vi "real time object finder single cam 4 way v2.2 EJA 10 31 2016.vi"() -> ()   [LabVIEW 2013]
doc: "The Low-Level Grab VI acquires images continuously and displays the images in an image control using low-level acquisition VIs. A grab is appropriate for high-speed applications in which you need to process only one image at a time."
uses:
  <vilib>/userdefined/High Color/IMAQdx.ctl
  <vilib>/vision/driver/IMAQdx.llb/IMAQdx Buffer Number Mode.ctl
  <vilib>/Utility/file.llb/Write To Spreadsheet File (I64).vi
  <vilib>/vision/driver/NI_Vision_Acquisition_Software.lvlib
  <resource>/objmgr/imaqdx.rc
  <vilib>/Analysis/NI_AALBase.lvlib
panel:
  in  "Rectangle":T1
  in  "fish size":i32=200
  out "y position histogram":T2(graph)={"X Values"=[445.05, 445.15, 445.25, 445.35, 445.45, 445.55, 445.65, 445.75, 445.85, 445.95], "Histogram: h(x)"=[161, 0, 0, 0, 0, 0, 0, 0, 0, 90]}
  out "x position histogram":T2(graph)={"X Values"=[585.0, 585.0, 585.0, 585.0, 585.0, 585.0, 585.0, 585.0, 585.0, 585.0], "Histogram: h(x)"=[0, 0, 0, 0, 0, 0, 0, 0, 0, 251]}
  in  "histogram \nbins":i32=10
  in  "always save\non stop\nimaging":bool=TRUE
  in  "acquisition \ntime (s)":i32=5
  in  "save for a \ndesignated \nperiod":bool=TRUE
  out "trajectory":cluster{i32[], i32[]}(graph)={[585, 585, 585, 585, 585, 585, 585, 585, 585, 585, 585, 585, 585, 585, 585, 585, 585, 585, 585, 585, 585, 585, 585, 585, 585, 585, 585, 585, 585, 585, 585, 585, 585, 585, 585, 585, 585, 585, 585, 585, 585, 585, 585, 585, 585, 585, 585, 585, 585, 585, 585, 585, 585, 585, 585, 585, 585, 585, 585, 585, 585, 585, 585, 585, 585, 585, 585, 585, 585, 585, 585, 585, 585, 585, 585, 585, 585, 585, 585, 585, 585, 585, 585, 585, 585, 585, 585, 585, 585, 585, 585, 585, 585, 585, 585, 585, 585, 585, 585, 585, 585, 585, 585, 585, 585, 585, 585, 585, 585, 585, 585, 585, 585, 585, 585, 585, 585, 585, 585, 585, 585, 585, 585, 585, 585, 585, 585, 585, 585, 585, 585, 585, 585, 585, 585, 585, 585, 585, 585, 585, 585, 585, 585, 585, 585, 585, 585, 585, 585, 585, 585, 585, 585, 585, 585, 585, 585, 585, 585, 585, 585, 585, 585, 585, 585, 585, 585, 585, 585, 585, 585, 585, 585, 585, 585, 585, 585, 585, 585, 585, 585, 585, 585, 585, 585, 585, 585, 585, 585, 585, 585, 585, 585, 585, 585, 585, 585, 585, 585, 585, 585, 585, 585, 585, 585, 585, 585, 585, 585, 585, 585, 585, 585, 585, 585, 585, 585, 585, 585, 585, 585, 585, 585, 585, 585, 585, 585, 585, 585, 585, 585, 585, 585, 585, 585, 585, 585, 585, 585, 585, 585, 585, 585, 585, 585, 585, 585, 585, 585, 585, 585], [446, 446, 445, 445, 446, 445, 446, 445, 445, 445, 446, 445, 445, 446, 445, 445, 445, 446, 446, 445, 445, 446, 446, 445, 446, 445, 445, 445, 445, 445, 445, 445, 446, 446, 446, 445, 445, 446, 446, 446, 445, 445, 445, 445, 446, 446, 445, 445, 445, 446, 446, 446, 445, 446, 445, 445, 445, 445, 445, 445, 445, 446, 445, 445, 445, 445, 446, 445, 445, 445, 446, 445, 445, 445, 446, 446, 446, 445, 445, 445, 446, 446, 445, 445, 446, 445, 445, 446, 445, 445, 446, 445, 445, 445, 446, 446, 446, 445, 445, 445, 445, 445, 445, 446, 446, 446, 446, 445, 445, 445, 445, 446, 445, 446, 446, 445, 445, 445, 445, 446, 445, 445, 445, 446, 446, 446, 446, 446, 445, 445, 445, 446, 445, 445, 445, 445, 446, 445, 445, 445, 445, 445, 445, 446, 445, 446, 446, 446, 445, 445, 445, 445, 445, 446, 445, 446, 445, 445, 446, 445, 446, 445, 445, 445, 445, 445, 446, 446, 446, 446, 446, 445, 445, 446, 445, 445, 446, 445, 445, 445, 445, 446, 445, 445, 445, 445, 445, 445, 445, 446, 445, 445, 445, 446, 445, 445, 445, 446, 446, 445, 446, 445, 445, 446, 446, 445, 446, 445, 445, 445, 445, 445, 445, 445, 446, 445, 445, 445, 446, 445, 446, 445, 446, 446, 445, 446, 445, 445, 446, 446, 445, 445, 445, 446, 445, 445, 446, 445, 446, 445, 445, 445, 445, 446, 445, 445, 445, 445, 446, 445, 446]}
  in  "save\nlast\nimage":bool=TRUE
  in  "stop no save":bool
  out "date stub assigned":string="_2016Y_10M_31D_13h_38m_14s"
  in  "Acquire\ndata":bool
  in  "Experimental stub":string="danio02"
  out "Saving":bool
  in  "save data":bool
  in  "save path":path=path "C:/danio_tracking/danio02_10_28_2016"
  in  "number\nformat (%.6f)":string="%.6f"
  in  "Marker\nText color":u32(colorbox)=16711680
  out "Multiplot":cluster{cluster{dbl, i32}[]}[](graph)=[{[{0.0, 585}, {0.02, 585}, {0.04, 585}, {0.06, 585}, {0.08, 585}, {0.1, 585}, {0.12, 585}, {0.14, 585}, {0.16, 585}, {0.18, 585}, {0.2, 585}, {0.22, 585}, {0.24, 585}, {0.26, 585}, {0.28, 585}, {0.3, 585}, {0.32, 585}, {0.34, 585}, {0.36, 585}, {0.38, 585}, {0.4, 585}, {0.42, 585}, {0.44, 585}, {0.461, 585}, {0.48, 585}, {0.5, 585}, {0.52, 585}, {0.541, 585}, {0.561, 585}, {0.58, 585}, {0.601, 585}, {0.62, 585}, {0.641, 585}, {0.661, 585}, {0.681, 585}, {0.701, 585}, {0.721, 585}, {0.741, 585}, {0.761, 585}, {0.781, 585}, {0.801, 585}, {0.821, 585}, {0.841, 585}, {0.861, 585}, {0.881, 585}, {0.901, 585}, {0.921, 585}, {0.941, 585}, {0.961, 585}, {0.981, 585}, {1.001, 585}, {1.021, 585}, {1.041, 585}, {1.061, 585}, {1.082, 585}, {1.102, 585}, {1.122, 585}, {1.142, 585}, {1.162, 585}, {1.182, 585}, {1.202, 585}, {1.222, 585}, {1.242, 585}, {1.263, 585}, {1.282, 585}, {1.302, 585}, {1.322, 585}, {1.342, 585}, {1.363, 585}, {1.382, 585}, {1.402, 585}, {1.422, 585}, {1.442, 585}, {1.463, 585}, {1.482, 585}, {1.502, 585}, {1.522, 585}, {1.542, 585}, {1.563, 585}, {1.582, 585}, {1.602, 585}, {1.623, 585}, {1.642, 585}, {1.663, 585}, {1.682, 585}, {1.703, 585}, {1.723, 585}, {1.743, 585}, {1.763, 585}, {1.783, 585}, {1.803, 585}, {1.823, 585}, {1.843, 585}, {1.863, 585}, {1.883, 585}, {1.903, 585}, {1.923, 585}, {1.943, 585}, {1.963, 585}, {1.983, 585}, {2.003, 585}, {2.023, 585}, {2.043, 585}, {2.063, 585}, {2.083, 585}, {2.103, 585}, {2.123, 585}, {2.143, 585}, {2.163, 585}, {2.183, 585}, {2.203, 585}, {2.223, 585}, {2.243, 585}, {2.263, 585}, {2.283, 585}, {2.303, 585}, {2.323, 585}, {2.343, 585}, {2.363, 585}, {2.383, 585}, {2.403, 585}, {2.423, 585}, {2.443, 585}, {2.463, 585}, {2.484, 585}, {2.503, 585}, {2.524, 585}, {2.544, 585}, {2.564, 585}, {2.584, 585}, {2.604, 585}, {2.624, 585}, {2.644, 585}, {2.664, 585}, {2.684, 585}, {2.705, 585}, {2.725, 585}, {2.745, 585}, {2.765, 585}, {2.784, 585}, {2.805, 585}, {2.825, 585}, {2.845, 585}, {2.865, 585}, {2.885, 585}, {2.905, 585}, {2.925, 585}, {2.945, 585}, {2.965, 585}, {2.985, 585}, {3.005, 585}, {3.025, 585}, {3.045, 585}, {3.065, 585}, {3.085, 585}, {3.105, 585}, {3.125, 585}, {3.145, 585}, {3.165, 585}, {3.185, 585}, {3.205, 585}, {3.225, 585}, {3.245, 585}, {3.265, 585}, {3.285, 585}, {3.305, 585}, {3.325, 585}, {3.345, 585}, {3.365, 585}, {3.385, 585}, {3.405, 585}, {3.425, 585}, {3.445, 585}, {3.465, 585}, {3.485, 585}, {3.505, 585}, {3.525, 585}, {3.545, 585}, {3.565, 585}, {3.585, 585}, {3.605, 585}, {3.625, 585}, {3.646, 585}, {3.665, 585}, {3.685, 585}, {3.705, 585}, {3.725, 585}, {3.747, 585}, {3.765, 585}, {3.786, 585}, {3.805, 585}, {3.825, 585}, {3.846, 585}, {3.865, 585}, {3.885, 585}, {3.907, 585}, {3.927, 585}, {3.947, 585}, {3.967, 585}, {3.987, 585}, {4.007, 585}, {4.027, 585}, {4.047, 585}, {4.067, 585}, {4.087, 585}, {4.107, 585}, {4.127, 585}, {4.147, 585}, {4.167, 585}, {4.187, 585}, {4.207, 585}, {4.227, 585}, {4.247, 585}, {4.267, 585}, {4.287, 585}, {4.307, 585}, {4.327, 585}, {4.347, 585}, {4.367, 585}, {4.387, 585}, {4.407, 585}, {4.427, 585}, {4.447, 585}, {4.467, 585}, {4.487, 585}, {4.507, 585}, {4.527, 585}, {4.547, 585}, {4.567, 585}, {4.587, 585}, {4.607, 585}, {4.627, 585}, {4.647, 585}, {4.667, 585}, {4.687, 585}, {4.707, 585}, {4.727, 585}, {4.748, 585}, {4.767, 585}, {4.787, 585}, {4.807, 585}, {4.828, 585}, {4.848, 585}, {4.867, 585}, {4.887, 585}, {4.907, 585}, {4.927, 585}, {4.948, 585}, {4.967, 585}, {4.988, 585}, {5.008, 585}]}, {[{0.0, 446}, {0.02, 446}, {0.04, 445}, {0.06, 445}, {0.08, 446}, {0.1, 445}, {0.12, 446}, {0.14, 445}, {0.16, 445}, {0.18, 445}, {0.2, 446}, {0.22, 445}, {0.24, 445}, {0.26, 446}, {0.28, 445}, {0.3, 445}, {0.32, 445}, {0.34, 446}, {0.36, 446}, {0.38, 445}, {0.4, 445}, {0.42, 446}, {0.44, 446}, {0.461, 445}, {0.48, 446}, {0.5, 445}, {0.52, 445}, {0.541, 445}, {0.561, 445}, {0.58, 445}, {0.601, 445}, {0.62, 445}, {0.641, 446}, {0.661, 446}, {0.681, 446}, {0.701, 445}, {0.721, 445}, {0.741, 446}, {0.761, 446}, {0.781, 446}, {0.801, 445}, {0.821, 445}, {0.841, 445}, {0.861, 445}, {0.881, 446}, {0.901, 446}, {0.921, 445}, {0.941, 445}, {0.961, 445}, {0.981, 446}, {1.001, 446}, {1.021, 446}, {1.041, 445}, {1.061, 446}, {1.082, 445}, {1.102, 445}, {1.122, 445}, {1.142, 445}, {1.162, 445}, {1.182, 445}, {1.202, 445}, {1.222, 446}, {1.242, 445}, {1.263, 445}, {1.282, 445}, {1.302, 445}, {1.322, 446}, {1.342, 445}, {1.363, 445}, {1.382, 445}, {1.402, 446}, {1.422, 445}, {1.442, 445}, {1.463, 445}, {1.482, 446}, {1.502, 446}, {1.522, 446}, {1.542, 445}, {1.563, 445}, {1.582, 445}, {1.602, 446}, {1.623, 446}, {1.642, 445}, {1.663, 445}, {1.682, 446}, {1.703, 445}, {1.723, 445}, {1.743, 446}, {1.763, 445}, {1.783, 445}, {1.803, 446}, {1.823, 445}, {1.843, 445}, {1.863, 445}, {1.883, 446}, {1.903, 446}, {1.923, 446}, {1.943, 445}, {1.963, 445}, {1.983, 445}, {2.003, 445}, {2.023, 445}, {2.043, 445}, {2.063, 446}, {2.083, 446}, {2.103, 446}, {2.123, 446}, {2.143, 445}, {2.163, 445}, {2.183, 445}, {2.203, 445}, {2.223, 446}, {2.243, 445}, {2.263, 446}, {2.283, 446}, {2.303, 445}, {2.323, 445}, {2.343, 445}, {2.363, 445}, {2.383, 446}, {2.403, 445}, {2.423, 445}, {2.443, 445}, {2.463, 446}, {2.484, 446}, {2.503, 446}, {2.524, 446}, {2.544, 446}, {2.564, 445}, {2.584, 445}, {2.604, 445}, {2.624, 446}, {2.644, 445}, {2.664, 445}, {2.684, 445}, {2.705, 445}, {2.725, 446}, {2.745, 445}, {2.765, 445}, {2.784, 445}, {2.805, 445}, {2.825, 445}, {2.845, 445}, {2.865, 446}, {2.885, 445}, {2.905, 446}, {2.925, 446}, {2.945, 446}, {2.965, 445}, {2.985, 445}, {3.005, 445}, {3.025, 445}, {3.045, 445}, {3.065, 446}, {3.085, 445}, {3.105, 446}, {3.125, 445}, {3.145, 445}, {3.165, 446}, {3.185, 445}, {3.205, 446}, {3.225, 445}, {3.245, 445}, {3.265, 445}, {3.285, 445}, {3.305, 445}, {3.325, 446}, {3.345, 446}, {3.365, 446}, {3.385, 446}, {3.405, 446}, {3.425, 445}, {3.445, 445}, {3.465, 446}, {3.485, 445}, {3.505, 445}, {3.525, 446}, {3.545, 445}, {3.565, 445}, {3.585, 445}, {3.605, 445}, {3.625, 446}, {3.646, 445}, {3.665, 445}, {3.685, 445}, {3.705, 445}, {3.725, 445}, {3.747, 445}, {3.765, 445}, {3.786, 446}, {3.805, 445}, {3.825, 445}, {3.846, 445}, {3.865, 446}, {3.885, 445}, {3.907, 445}, {3.927, 445}, {3.947, 446}, {3.967, 446}, {3.987, 445}, {4.007, 446}, {4.027, 445}, {4.047, 445}, {4.067, 446}, {4.087, 446}, {4.107, 445}, {4.127, 446}, {4.147, 445}, {4.167, 445}, {4.187, 445}, {4.207, 445}, {4.227, 445}, {4.247, 445}, {4.267, 445}, {4.287, 446}, {4.307, 445}, {4.327, 445}, {4.347, 445}, {4.367, 446}, {4.387, 445}, {4.407, 446}, {4.427, 445}, {4.447, 446}, {4.467, 446}, {4.487, 445}, {4.507, 446}, {4.527, 445}, {4.547, 445}, {4.567, 446}, {4.587, 446}, {4.607, 445}, {4.627, 445}, {4.647, 445}, {4.667, 446}, {4.687, 445}, {4.707, 445}, {4.727, 446}, {4.748, 445}, {4.767, 446}, {4.787, 445}, {4.807, 445}, {4.828, 445}, {4.848, 445}, {4.867, 446}, {4.887, 445}, {4.907, 445}, {4.927, 445}, {4.948, 445}, {4.967, 446}, {4.988, 445}, {5.008, 446}]}]
  out "FPS":i32=50
  out "time (s)":dbl[](array[numeric])=[0.0, 0.02, 0.04, 0.06, 0.08, 0.1, 0.12, 0.14, 0.16, 0.18, 0.2, 0.22, 0.24, 0.26, 0.28, 0.3, 0.32, 0.34, 0.36, 0.38, 0.4, 0.42, 0.44, 0.461, 0.48, 0.5, 0.52, 0.541, 0.561, 0.58, 0.601, 0.62, 0.641, 0.661, 0.681, 0.701, 0.721, 0.741, 0.761, 0.781, 0.801, 0.821, 0.841, 0.861, 0.881, 0.901, 0.921, 0.941, 0.961, 0.981, 1.001, 1.021, 1.041, 1.061, 1.082, 1.102, 1.122, 1.142, 1.162, 1.182, 1.202, 1.222, 1.242, 1.263, 1.282, 1.302, 1.322, 1.342, 1.363, 1.382, 1.402, 1.422, 1.442, 1.463, 1.482, 1.502, 1.522, 1.542, 1.563, 1.582, 1.602, 1.623, 1.642, 1.663, 1.682, 1.703, 1.723, 1.743, 1.763, 1.783, 1.803, 1.823, 1.843, 1.863, 1.883, 1.903, 1.923, 1.943, 1.963, 1.983, 2.003, 2.023, 2.043, 2.063, 2.083, 2.103, 2.123, 2.143, 2.163, 2.183, 2.203, 2.223, 2.243, 2.263, 2.283, 2.303, 2.323, 2.343, 2.363, 2.383, 2.403, 2.423, 2.443, 2.463, 2.484, 2.503, 2.524, 2.544, 2.564, 2.584, 2.604, 2.624, 2.644, 2.664, 2.684, 2.705, 2.725, 2.745, 2.765, 2.784, 2.805, 2.825, 2.845, 2.865, 2.885, 2.905, 2.925, 2.945, 2.965, 2.985, 3.005, 3.025, 3.045, 3.065, 3.085, 3.105, 3.125, 3.145, 3.165, 3.185, 3.205, 3.225, 3.245, 3.265, 3.285, 3.305, 3.325, 3.345, 3.365, 3.385, 3.405, 3.425, 3.445, 3.465, 3.485, 3.505, 3.525, 3.545, 3.565, 3.585, 3.605, 3.625, 3.646, 3.665, 3.685, 3.705, 3.725, 3.747, 3.765, 3.786, 3.805, 3.825, 3.846, 3.865, 3.885, 3.907, 3.927, 3.947, 3.967, 3.987, 4.007, 4.027, 4.047, 4.067, 4.087, 4.107, 4.127, 4.147, 4.167, 4.187, 4.207, 4.227, 4.247, 4.267, 4.287, 4.307, 4.327, 4.347, 4.367, 4.387, 4.407, 4.427, 4.447, 4.467, 4.487, 4.507, 4.527, 4.547, 4.567, 4.587, 4.607, 4.627, 4.647, 4.667, 4.687, 4.707, 4.727, 4.748, 4.767, 4.787, 4.807, 4.828, 4.848, 4.867, 4.887, 4.907, 4.927, 4.948, 4.967, 4.988, 5.008] format="%.3f"
  in  "Origin":cluster{"X":i32, "Y":i32}
  out "Y position vs time":cluster{dbl[], i32[]}(graph)={[0.0, 0.02, 0.04, 0.06, 0.08, 0.1, 0.12, 0.14, 0.16, 0.18, 0.2, 0.22, 0.24, 0.26, 0.28, 0.3, 0.32, 0.34, 0.36, 0.38, 0.4, 0.42, 0.44, 0.461, 0.48, 0.5, 0.52, 0.541, 0.561, 0.58, 0.601, 0.62, 0.641, 0.661, 0.681, 0.701, 0.721, 0.741, 0.761, 0.781, 0.801, 0.821, 0.841, 0.861, 0.881, 0.901, 0.921, 0.941, 0.961, 0.981, 1.001, 1.021, 1.041, 1.061, 1.082, 1.102, 1.122, 1.142, 1.162, 1.182, 1.202, 1.222, 1.242, 1.263, 1.282, 1.302, 1.322, 1.342, 1.363, 1.382, 1.402, 1.422, 1.442, 1.463, 1.482, 1.502, 1.522, 1.542, 1.563, 1.582, 1.602, 1.623, 1.642, 1.663, 1.682, 1.703, 1.723, 1.743, 1.763, 1.783, 1.803, 1.823, 1.843, 1.863, 1.883, 1.903, 1.923, 1.943, 1.963, 1.983, 2.003, 2.023, 2.043, 2.063, 2.083, 2.103, 2.123, 2.143, 2.163, 2.183, 2.203, 2.223, 2.243, 2.263, 2.283, 2.303, 2.323, 2.343, 2.363, 2.383, 2.403, 2.423, 2.443, 2.463, 2.484, 2.503, 2.524, 2.544, 2.564, 2.584, 2.604, 2.624, 2.644, 2.664, 2.684, 2.705, 2.725, 2.745, 2.765, 2.784, 2.805, 2.825, 2.845, 2.865, 2.885, 2.905, 2.925, 2.945, 2.965, 2.985, 3.005, 3.025, 3.045, 3.065, 3.085, 3.105, 3.125, 3.145, 3.165, 3.185, 3.205, 3.225, 3.245, 3.265, 3.285, 3.305, 3.325, 3.345, 3.365, 3.385, 3.405, 3.425, 3.445, 3.465, 3.485, 3.505, 3.525, 3.545, 3.565, 3.585, 3.605, 3.625, 3.646, 3.665, 3.685, 3.705, 3.725, 3.747, 3.765, 3.786, 3.805, 3.825, 3.846, 3.865, 3.885, 3.907, 3.927, 3.947, 3.967, 3.987, 4.007, 4.027, 4.047, 4.067, 4.087, 4.107, 4.127, 4.147, 4.167, 4.187, 4.207, 4.227, 4.247, 4.267, 4.287, 4.307, 4.327, 4.347, 4.367, 4.387, 4.407, 4.427, 4.447, 4.467, 4.487, 4.507, 4.527, 4.547, 4.567, 4.587, 4.607, 4.627, 4.647, 4.667, 4.687, 4.707, 4.727, 4.748, 4.767, 4.787, 4.807, 4.828, 4.848, 4.867, 4.887, 4.907, 4.927, 4.948, 4.967, 4.988, 5.008], [446, 446, 445, 445, 446, 445, 446, 445, 445, 445, 446, 445, 445, 446, 445, 445, 445, 446, 446, 445, 445, 446, 446, 445, 446, 445, 445, 445, 445, 445, 445, 445, 446, 446, 446, 445, 445, 446, 446, 446, 445, 445, 445, 445, 446, 446, 445, 445, 445, 446, 446, 446, 445, 446, 445, 445, 445, 445, 445, 445, 445, 446, 445, 445, 445, 445, 446, 445, 445, 445, 446, 445, 445, 445, 446, 446, 446, 445, 445, 445, 446, 446, 445, 445, 446, 445, 445, 446, 445, 445, 446, 445, 445, 445, 446, 446, 446, 445, 445, 445, 445, 445, 445, 446, 446, 446, 446, 445, 445, 445, 445, 446, 445, 446, 446, 445, 445, 445, 445, 446, 445, 445, 445, 446, 446, 446, 446, 446, 445, 445, 445, 446, 445, 445, 445, 445, 446, 445, 445, 445, 445, 445, 445, 446, 445, 446, 446, 446, 445, 445, 445, 445, 445, 446, 445, 446, 445, 445, 446, 445, 446, 445, 445, 445, 445, 445, 446, 446, 446, 446, 446, 445, 445, 446, 445, 445, 446, 445, 445, 445, 445, 446, 445, 445, 445, 445, 445, 445, 445, 446, 445, 445, 445, 446, 445, 445, 445, 446, 446, 445, 446, 445, 445, 446, 446, 445, 446, 445, 445, 445, 445, 445, 445, 445, 446, 445, 445, 445, 446, 445, 446, 445, 446, 446, 445, 446, 445, 445, 446, 446, 445, 445, 445, 446, 445, 445, 446, 445, 446, 445, 445, 445, 445, 446, 445, 445, 445, 445, 446, 445, 446]}
  out "X position vs time":cluster{dbl[], i32[]}(graph)={[0.0, 0.02, 0.04, 0.06, 0.08, 0.1, 0.12, 0.14, 0.16, 0.18, 0.2, 0.22, 0.24, 0.26, 0.28, 0.3, 0.32, 0.34, 0.36, 0.38, 0.4, 0.42, 0.44, 0.461, 0.48, 0.5, 0.52, 0.541, 0.561, 0.58, 0.601, 0.62, 0.641, 0.661, 0.681, 0.701, 0.721, 0.741, 0.761, 0.781, 0.801, 0.821, 0.841, 0.861, 0.881, 0.901, 0.921, 0.941, 0.961, 0.981, 1.001, 1.021, 1.041, 1.061, 1.082, 1.102, 1.122, 1.142, 1.162, 1.182, 1.202, 1.222, 1.242, 1.263, 1.282, 1.302, 1.322, 1.342, 1.363, 1.382, 1.402, 1.422, 1.442, 1.463, 1.482, 1.502, 1.522, 1.542, 1.563, 1.582, 1.602, 1.623, 1.642, 1.663, 1.682, 1.703, 1.723, 1.743, 1.763, 1.783, 1.803, 1.823, 1.843, 1.863, 1.883, 1.903, 1.923, 1.943, 1.963, 1.983, 2.003, 2.023, 2.043, 2.063, 2.083, 2.103, 2.123, 2.143, 2.163, 2.183, 2.203, 2.223, 2.243, 2.263, 2.283, 2.303, 2.323, 2.343, 2.363, 2.383, 2.403, 2.423, 2.443, 2.463, 2.484, 2.503, 2.524, 2.544, 2.564, 2.584, 2.604, 2.624, 2.644, 2.664, 2.684, 2.705, 2.725, 2.745, 2.765, 2.784, 2.805, 2.825, 2.845, 2.865, 2.885, 2.905, 2.925, 2.945, 2.965, 2.985, 3.005, 3.025, 3.045, 3.065, 3.085, 3.105, 3.125, 3.145, 3.165, 3.185, 3.205, 3.225, 3.245, 3.265, 3.285, 3.305, 3.325, 3.345, 3.365, 3.385, 3.405, 3.425, 3.445, 3.465, 3.485, 3.505, 3.525, 3.545, 3.565, 3.585, 3.605, 3.625, 3.646, 3.665, 3.685, 3.705, 3.725, 3.747, 3.765, 3.786, 3.805, 3.825, 3.846, 3.865, 3.885, 3.907, 3.927, 3.947, 3.967, 3.987, 4.007, 4.027, 4.047, 4.067, 4.087, 4.107, 4.127, 4.147, 4.167, 4.187, 4.207, 4.227, 4.247, 4.267, 4.287, 4.307, 4.327, 4.347, 4.367, 4.387, 4.407, 4.427, 4.447, 4.467, 4.487, 4.507, 4.527, 4.547, 4.567, 4.587, 4.607, 4.627, 4.647, 4.667, 4.687, 4.707, 4.727, 4.748, 4.767, 4.787, 4.807, 4.828, 4.848, 4.867, 4.887, 4.907, 4.927, 4.948, 4.967, 4.988, 5.008], [585, 585, 585, 585, 585, 585, 585, 585, 585, 585, 585, 585, 585, 585, 585, 585, 585, 585, 585, 585, 585, 585, 585, 585, 585, 585, 585, 585, 585, 585, 585, 585, 585, 585, 585, 585, 585, 585, 585, 585, 585, 585, 585, 585, 585, 585, 585, 585, 585, 585, 585, 585, 585, 585, 585, 585, 585, 585, 585, 585, 585, 585, 585, 585, 585, 585, 585, 585, 585, 585, 585, 585, 585, 585, 585, 585, 585, 585, 585, 585, 585, 585, 585, 585, 585, 585, 585, 585, 585, 585, 585, 585, 585, 585, 585, 585, 585, 585, 585, 585, 585, 585, 585, 585, 585, 585, 585, 585, 585, 585, 585, 585, 585, 585, 585, 585, 585, 585, 585, 585, 585, 585, 585, 585, 585, 585, 585, 585, 585, 585, 585, 585, 585, 585, 585, 585, 585, 585, 585, 585, 585, 585, 585, 585, 585, 585, 585, 585, 585, 585, 585, 585, 585, 585, 585, 585, 585, 585, 585, 585, 585, 585, 585, 585, 585, 585, 585, 585, 585, 585, 585, 585, 585, 585, 585, 585, 585, 585, 585, 585, 585, 585, 585, 585, 585, 585, 585, 585, 585, 585, 585, 585, 585, 585, 585, 585, 585, 585, 585, 585, 585, 585, 585, 585, 585, 585, 585, 585, 585, 585, 585, 585, 585, 585, 585, 585, 585, 585, 585, 585, 585, 585, 585, 585, 585, 585, 585, 585, 585, 585, 585, 585, 585, 585, 585, 585, 585, 585, 585, 585, 585, 585, 585, 585, 585, 585, 585, 585, 585, 585, 585]}
  in  "Pixel intensity\nthreshold":i32=65
  in  "Row min":i32=136
  in  "Row max":i32=630
  in  "Column min":i32=120
  in  "Column max":i32=1027
  out "X positions\ncamera 1\n(image \ncoordinates)":i32[](array[numeric])=[585, 585, 585, 585, 585, 585, 585, 585, 585, 585, 585, 585, 585, 585, 585, 585, 585, 585, 585, 585, 585, 585, 585, 585, 585, 585, 585, 585, 585, 585, 585, 585, 585, 585, 585, 585, 585, 585, 585, 585, 585, 585, 585, 585, 585, 585, 585, 585, 585, 585, 585, 585, 585, 585, 585, 585, 585, 585, 585, 585, 585, 585, 585, 585, 585, 585, 585, 585, 585, 585, 585, 585, 585, 585, 585, 585, 585, 585, 585, 585, 585, 585, 585, 585, 585, 585, 585, 585, 585, 585, 585, 585, 585, 585, 585, 585, 585, 585, 585, 585, 585, 585, 585, 585, 585, 585, 585, 585, 585, 585, 585, 585, 585, 585, 585, 585, 585, 585, 585, 585, 585, 585, 585, 585, 585, 585, 585, 585, 585, 585, 585, 585, 585, 585, 585, 585, 585, 585, 585, 585, 585, 585, 585, 585, 585, 585, 585, 585, 585, 585, 585, 585, 585, 585, 585, 585, 585, 585, 585, 585, 585, 585, 585, 585, 585, 585, 585, 585, 585, 585, 585, 585, 585, 585, 585, 585, 585, 585, 585, 585, 585, 585, 585, 585, 585, 585, 585, 585, 585, 585, 585, 585, 585, 585, 585, 585, 585, 585, 585, 585, 585, 585, 585, 585, 585, 585, 585, 585, 585, 585, 585, 585, 585, 585, 585, 585, 585, 585, 585, 585, 585, 585, 585, 585, 585, 585, 585, 585, 585, 585, 585, 585, 585, 585, 585, 585, 585, 585, 585, 585, 585, 585, 585, 585, 585, 585, 585, 585, 585, 585, 585]
  out "Y positions camera 1 \n(image \ncoordinates)":i32[](array[numeric])=[446, 446, 445, 445, 446, 445, 446, 445, 445, 445, 446, 445, 445, 446, 445, 445, 445, 446, 446, 445, 445, 446, 446, 445, 446, 445, 445, 445, 445, 445, 445, 445, 446, 446, 446, 445, 445, 446, 446, 446, 445, 445, 445, 445, 446, 446, 445, 445, 445, 446, 446, 446, 445, 446, 445, 445, 445, 445, 445, 445, 445, 446, 445, 445, 445, 445, 446, 445, 445, 445, 446, 445, 445, 445, 446, 446, 446, 445, 445, 445, 446, 446, 445, 445, 446, 445, 445, 446, 445, 445, 446, 445, 445, 445, 446, 446, 446, 445, 445, 445, 445, 445, 445, 446, 446, 446, 446, 445, 445, 445, 445, 446, 445, 446, 446, 445, 445, 445, 445, 446, 445, 445, 445, 446, 446, 446, 446, 446, 445, 445, 445, 446, 445, 445, 445, 445, 446, 445, 445, 445, 445, 445, 445, 446, 445, 446, 446, 446, 445, 445, 445, 445, 445, 446, 445, 446, 445, 445, 446, 445, 446, 445, 445, 445, 445, 445, 446, 446, 446, 446, 446, 445, 445, 446, 445, 445, 446, 445, 445, 445, 445, 446, 445, 445, 445, 445, 445, 445, 445, 446, 445, 445, 445, 446, 445, 445, 445, 446, 446, 445, 446, 445, 445, 446, 446, 445, 446, 445, 445, 445, 445, 445, 445, 445, 446, 445, 445, 445, 446, 445, 446, 445, 446, 446, 445, 446, 445, 445, 446, 446, 445, 445, 445, 446, 445, 445, 446, 445, 446, 445, 445, 445, 445, 446, 445, 445, 445, 445, 446, 445, 446]
  out "LIVE":bool
  in  "stop":bool
  out "Camera backlog":i32(slide)=-1 scale=0.0..50.0
  in  "IMAQdx Device Camera":T3="cam2"
  in  "Buffers Camera 1":u32=50
  out "Image":T4(plugin-control)
  # "PROGRAM INFO\n\nThis program finds the\nfirst pixel below the \nuser threshold in\nthe user specified\nROI below"
  # "Camera search ROI"
  # "Data acquisition \nsettings"
  # "issues\n\nHow do we know if frames \nare dropped?\n\nProbably will need to save data\nin sections to an open file\n\nCould have a sliding ROI based\non previous trailing edge position\n\nCould process each data chunk\nseparately to avoid frame dropping\nissues.  I.e. if you write every 1000\npoints, then in post processing only\nprocess 1000 at a time."
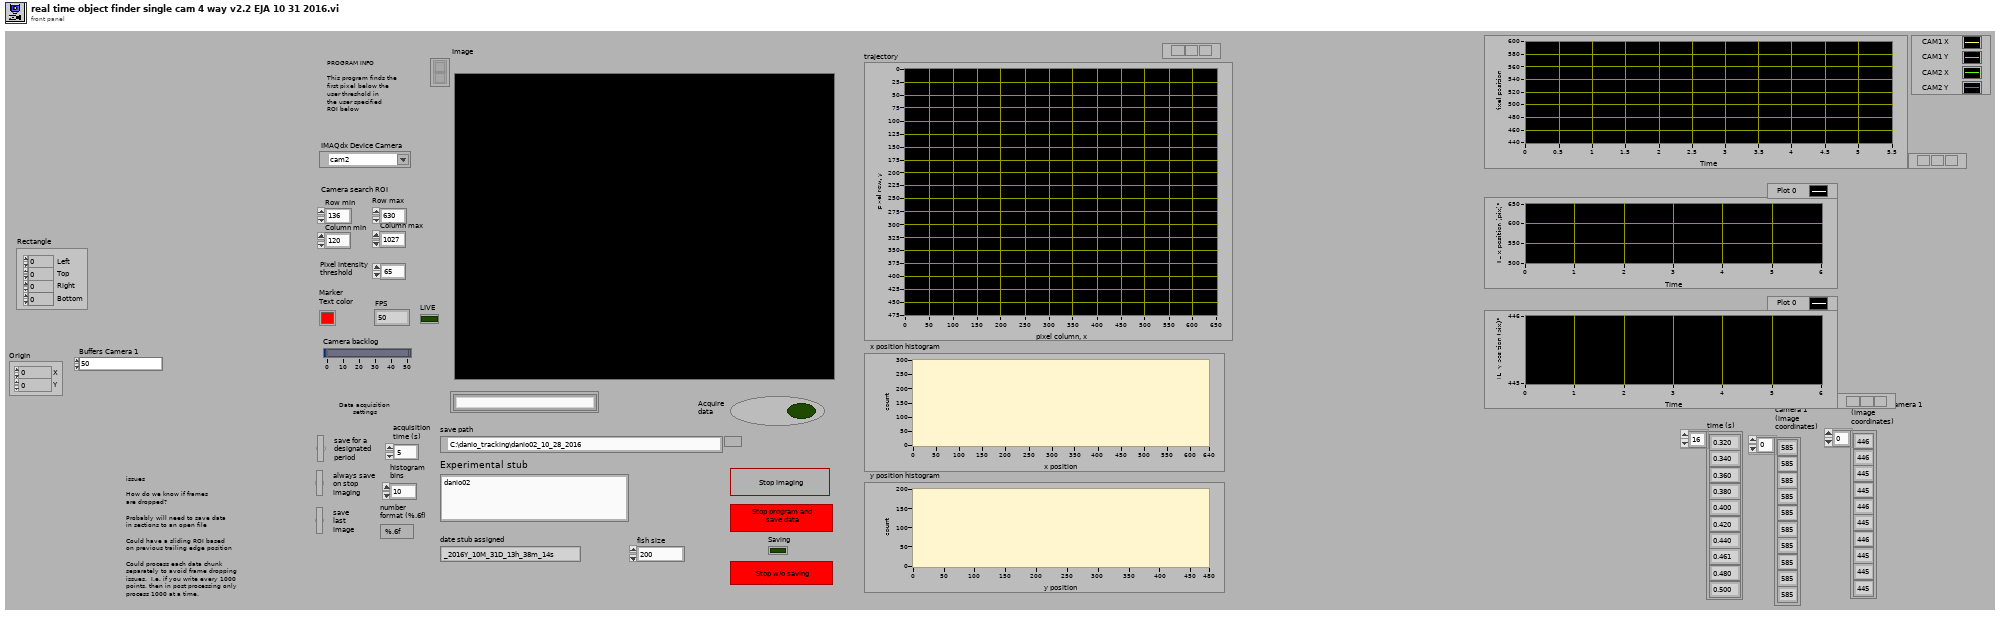
[diagram p1: front panel]
types:
  T1 = cluster{"Left":i32, "Top":i32, "Right":i32, "Bottom":i32}
  T2 = cluster{"X Values":dbl[], "Histogram: h(x)":i32[]}
  T3 = typedef "IMAQdx.ctl" = refnum<k21>
  T4 = typedef "IMAQ Image.ctl" = refnum<image>
  T5 = typedef "NI_Vision_Acquisition_Software.lvlib/IMAQdx Buffer Number Mode.ctl" = enum32{"Next", "Last", "Buffer Number"}
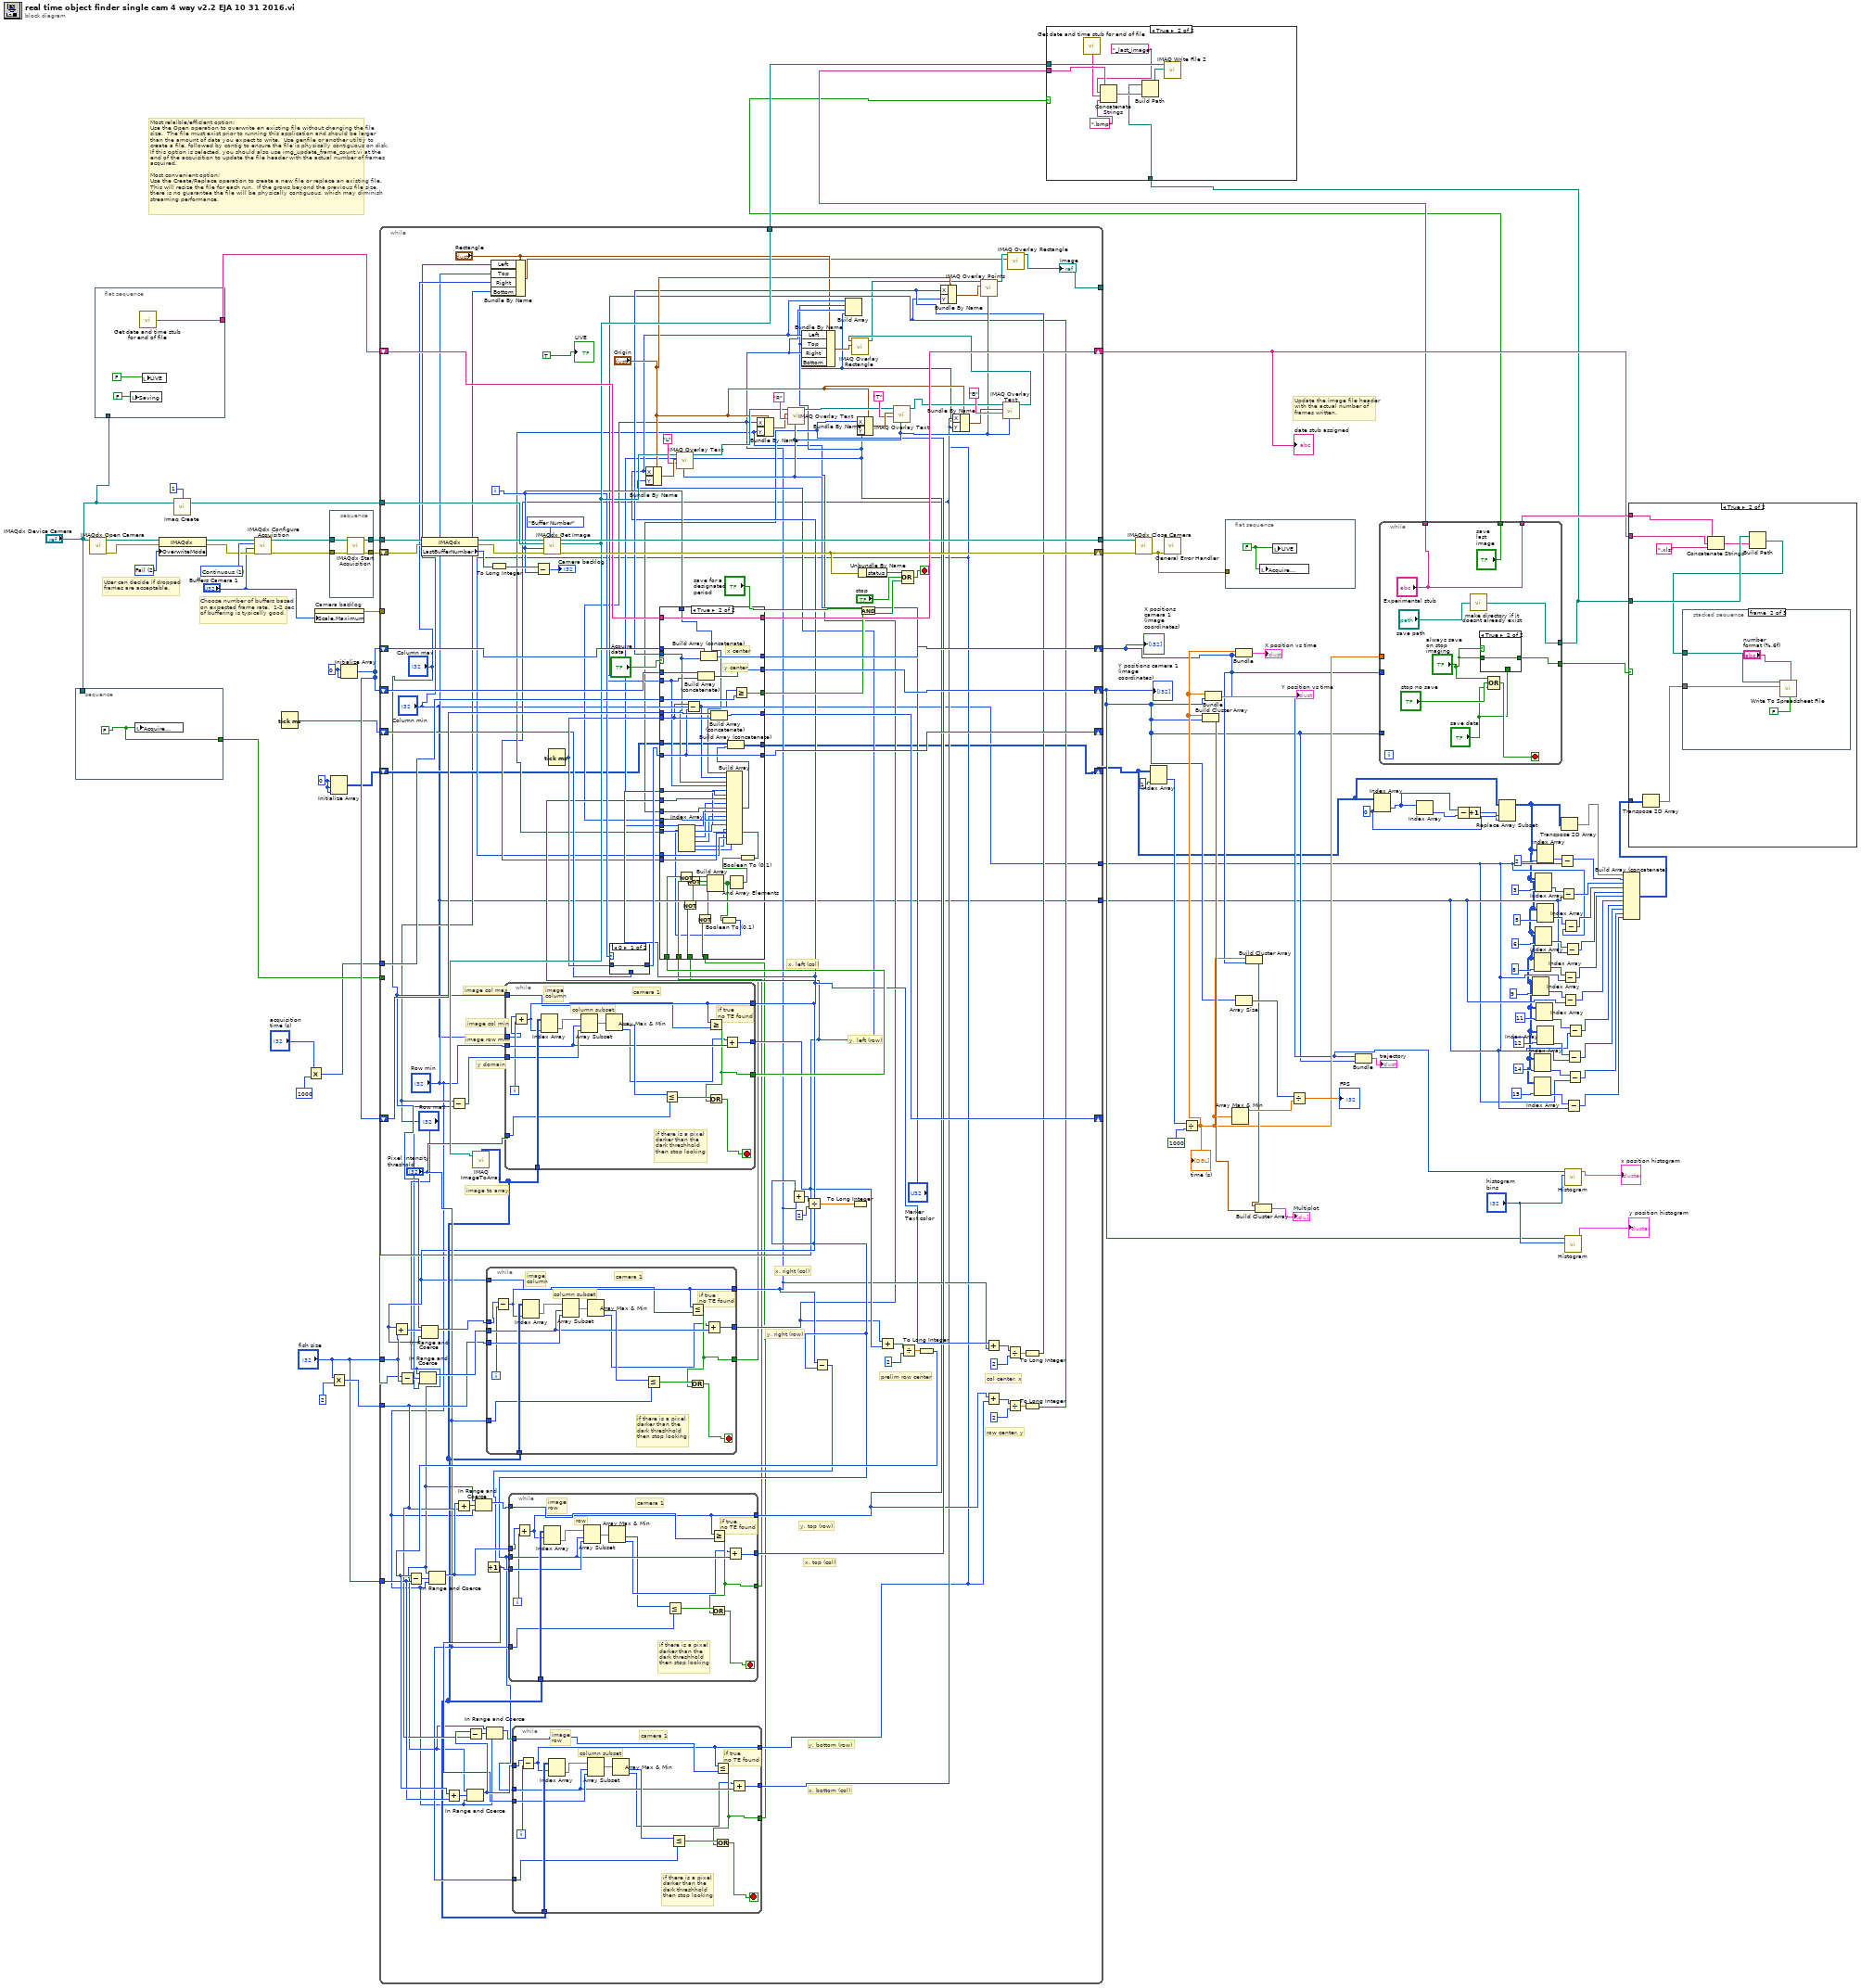
[diagram p0: block diagram]
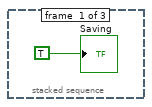
[diagram p4: hidden frame]
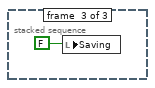
[diagram p5: hidden frame]
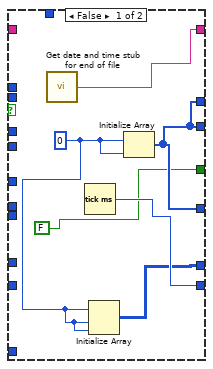
[diagram p8: hidden frame]
diagram:
  w37 = 0
  w45 = 0
  w70 = 0
  w90 = u32 2 items=["Get Oldest"=0, "Fail"=2, "Get Newest"=3] ("OverwriteMode")
  w96 = u32 1 items=["One Shot", "Continuous"] ("Continuous ?")
  # "Update the image file header with the actual number of frames written."
  # "Choose number of buffers based on expected frame rate.  1-2 sec of buffering is typically good."
  # "User can decide if dropped frames are acceptable."
  # "Most relaible/efficient option:\nUse the Open operation to overwrite an existing file without changing the file size.  The file must exist prior to running this application and should be larger than the amount of data you expect to write.  Use genfile or another utiltiy to create a file, followed by contig to ensure the file is physically contiguous on disk.  If this option is selected, you should also use img_update_frame_count.vi at the end of the acquisition to update the file header with the actual number of frames acquired. \n\nMost convenient option:\nUse the Create/Replace operation to create a new file or replace an existing file. This will resize the file for each run.  If the grows beyond the previous file size, there is no guarantee the file will be physically contiguous, which may diminish streaming performance."
  n1 = stacked-sequence {
    tunnel: "IMAQdx Device Camera" -> [_]
    tunnel: [w98] -> w60
    frame #0 {
      w98 = FALSE
      n2 = local write "Acquire\ndata"(w98) -> ()
    }
  }
  n3 = call <vilib>:"IMAQdx Open Camera.vi"("Session In"="IMAQdx Device Camera") -> ("error out"=w86:errorcluster, "Session Out"=w85:T3)  [unwired: 2 in, 7 out]
  n4 = flat-sequence {
    tunnel: "IMAQdx Device Camera" -> [_]
    tunnel: [w99] -> w69
    frame #0 {
      n5 = local write "Saving"(FALSE) -> ()
      n6 = call <userlib>:"Get date and time stub for end of file.vi"() -> ("date and time stub"=w99:string)
      n7 = local write "LIVE"(FALSE) -> ()
    }
  }
  n8 = property class="IMAQdx"(reference=w85, error in=w86, "OverwriteMode"=w90) -> (reference out=w88:T3, error out=w87:errorcluster)
  n9 = call "Imaq Create"("Border Size"=1, "Image Name"="IMAQdx Device Camera") -> ("New Image"=w97:T4)  [unwired: 2 in, 2 out]
  n10 = call <vilib>:"IMAQdx Configure Acquisition.vi"("error in"=w87, "Number of Buffers"="Buffers Camera 1", "Continuous?"=w96, "Session In"=w88) -> ("error out"=w82:errorcluster, "Session Out"=w89:T3)  [unwired: 6 out]
  n11 = Tick Count (ms)() -> (millisecond timer value=w54:u32)
  n12 = Multiply(x="acquisition \ntime (s)", y=1000) -> (x*y=w55:i32)
  n13 = property on="Camera backlog" class="Slide (strict)"("Scale.Maximum"="Buffers Camera 1") -> (error out=w84:errorcluster)  [unwired: 2 in, 1 out]
  n14 = stacked-sequence {
    tunnel: [w105] -> w95
    tunnel: [w104] -> w94
    tunnel: w89 -> [w103]
    tunnel: w82 -> [w102]
    frame #0 {
      n15 = call <vilib>:"IMAQdx Start Acquisition.vi"("error in"=w102, "Session In"=w103) -> ("error out"=w105:errorcluster, "Session Out"=w104:T3)  [unwired: 8 out]
    }
  }
  n16 = Initialize Array(w45, w45, w45) -> (w44:i32[][])
  n17 = Multiply(x="fish size", y=2) -> (x*y=w47:i32)
  n18 = Initialize Array(w70, w70) -> (w67:i32[])
  n19 = while {
    tunnel: [w208] -> w92
    tunnel: w94 -> [w211]
    tunnel: w97 -> [w209]
    tunnel: [w109] -> _
    shift-right: [w207] -> w91
    shift-left: w95 -> [w210]
    tunnel: w84 -> [_]
    shift-right: [w194] -> w53
    shift-left: w67 -> [w193]
    shift-right: [w192] -> w49
    shift-left: w67 -> [w191]
    shift-right: [w190] -> _
    shift-left: w67 -> [w189]
    shift-right: [w187] -> w68
    shift-left: w69 -> [w188]
    tunnel: [w185] -> w65
    tunnel: w60 -> [_]
    shift-right: [w184] -> _
    shift-left: w54 -> [w176]
    tunnel: w55 -> [w183]
    tunnel: "fish size" -> [w173]
    tunnel: w47 -> [w149]
    tunnel: "fish size" -> [w152]
    shift-right: [w118] -> w39
    shift-left: w44 -> [w119]
    tunnel: ["Row min"] -> w5
    tunnel: ["Column min"] -> w4
    i -> [w179]
    stop <- w213 stop-if-true
    # "x, top (col)"
    # "y, top (row)"
    # "row center, y"
    # "col center, x"
    # "y, bottom (row)"
    # "x, bottom (col)"
    # "prelim row center"
    # "x, right (col)"
    # "y, right (row)"
    # "image col min"
    # "image col max"
    # "image row min"
    # "y, left (row)"
    # "x, left (col)"
    # "y domain"
    # "image to array"
    n20 = property class="IMAQdx"(reference=w211, error in=w210) -> (reference out=w204:T3, error out=w205:errorcluster, "LastBufferNumber"=w201:u32)
    n21 = Subtract(x="Row max", y="Row min") -> (x-y=w196:i32)
    n22 = To Long Integer(number=w201) -> (32bit integer=w200:i32)
    n23 = Bundle By Name(cluster="Rectangle", "Left"="Column min", "Top"="Row min", "Right"="Column max", "Bottom"="Row max") -> (w108:T1)
    n24 = Subtract(x=w200, y=w179) -> (x-y=→"Camera backlog":i32)
    n25 = call <vilib>:"IMAQdx Get Image.vi"("Buffer Number Mode (Next)"=IMAQdx_Buffer_Number_Mode."Buffer Number", "error in"=w205, "Buffer Number In"=w179, "Image In"=w209, "Session In"=w204) -> ("error out"=w207:errorcluster, "Image Out"=w185:T4, "Session Out"=w208:T3)  [unwired: 1 in, 3 out]
    n26 = call "IMAQ ImageToArray"("Image"=w185) -> ("Image Pixels (U8)"=w144:u8[][])  [unwired: 2 in, 5 out]
    n27 = while {
      tunnel: "Row min" -> [w321]
      tunnel: [w320] -> w127
      tunnel: [w322] -> w126
      tunnel: w196 -> [w324]
      tunnel: w144 -> [w326]
      tunnel: "Column max" -> [w312]
      tunnel: "Column min" -> [w313]
      tunnel: [w317] -> w186
      tunnel: "Pixel intensity\nthreshold" -> [w315]
      i -> [w314]
      stop <- w318 stop-if-true
      # "if true\nno TE found"
      # "camera 1"
      # "if there is a pixel\ndarker than the\ndark threshhold\nthen stop looking"
      # "column subset"
      # "image\ncolumn"
      n28 = Add(x=w313, y=w314) -> (x+y=w320:i32)
      n29 = Index Array(array=w326, index (col)=w320) -> (element=w325:u8[])  [unwired: 1 in]
      n30 = Array Subset(array=w325, index=w321, length=w324) -> (w323:u8[])
      n31 = Array Max & Min(array=w323) -> (min value=w327:u8, min index (indices)=w316:i32)  [unwired: 2 out]
      n32 = Less Or Equal?(x=w327, y=w315) -> (x <= y?=w319:bool)
      n33 = Greater Or Equal?(x=w320, y=w312) -> (x >= y?=w317:bool)
      n34 = Or(x=w319, y=w317) -> (x .or. y?=w318:bool)
      n35 = Add(x=w316, y=w321) -> (x+y=w322:i32)
    }
    n36 = Add(x=w127, y=w173) -> (x+y=w175:i32)
    n37 = Subtract(x=w126, y=w173) -> (x-y=w172:i32)
    n38 = In Range and Coerce(upper limit="Row max", x=w172, lower limit="Row min") -> (coerced(x)=w171:i32)  [unwired: 1 out]
    n39 = In Range and Coerce(upper limit="Column max", x=w175, lower limit=w127) -> (coerced(x)=w174:i32)  [unwired: 1 out]
    n40 = while {
      tunnel: w171 -> [w255]
      tunnel: [w254] -> w124
      tunnel: [w256] -> w122
      tunnel: w149 -> [w258]
      tunnel: w144 -> [w260]
      tunnel: w127 -> [w246]
      tunnel: w174 -> [w247]
      tunnel: [w251] -> w116
      tunnel: "Pixel intensity\nthreshold" -> [w249]
      i -> [w248]
      stop <- w252 stop-if-true
      # "if true\nno TE found"
      # "camera 1"
      # "if there is a pixel\ndarker than the\ndark threshhold\nthen stop looking"
      # "column subset"
      # "image\ncolumn"
      n41 = Subtract(x=w247, y=w248) -> (x-y=w254:i32)
      n42 = Index Array(array=w260, index (col)=w254) -> (element=w259:u8[])  [unwired: 1 in]
      n43 = Array Subset(array=w259, index=w255, length=w258) -> (w257:u8[])
      n44 = Array Max & Min(array=w257) -> (min value=w261:u8, min index (indices)=w250:i32)  [unwired: 2 out]
      n45 = Less Or Equal?(x=w261, y=w249) -> (x <= y?=w253:bool)
      n46 = Less Or Equal?(x=w254, y=w246) -> (x <= y?=w251:bool)
      n47 = Or(x=w253, y=w251) -> (x .or. y?=w252:bool)
      n48 = Add(x=w250, y=w255) -> (x+y=w256:i32)
    }
    n49 = Tick Count (ms)() -> (millisecond timer value=w178:u32)
    n50 = case shown="0" w179 {
      tunnel: w178 -> [w262 _]
      tunnel: [w262 w263] -> w177
      tunnel: w176 -> [_ w263]
      frame 0 {
      }
      frame 1, Default {
      }
    }
    n51 = Bundle By Name(cluster="Origin", "X"=w127, "Y"=w126) -> (w198:cluster{"X":i32, "Y":i32})
    n52 = call "IMAQ Overlay Text"("Text Color (black)"="Marker\nText color", "String"="L", "Origin"=w198, "Image"=w185) -> ("Image Out"=w168:T4)  [unwired: 4 in, 3 out]
    n53 = Bundle By Name(cluster="Origin", "X"=w124, "Y"=w122) -> (w169:cluster{"X":i32, "Y":i32})
    n54 = call "IMAQ Overlay Text"("Text Color (black)"="Marker\nText color", "String"="R", "Origin"=w169, "Image"=w168) -> ("Image Out"=w155:T4)  [unwired: 4 in, 3 out]
    n55 = Add(x=w127, y=w124) -> (x+y=w167:i32)
    n56 = Divide(x=w167, y=2) -> (x/y=w165:dbl)
    n57 = Subtract(x=w124, y=w127) -> (x-y=w147:i32)
    n58 = Increment(x=w147) -> (x+1=w146:i32)
    n59 = To Long Integer(number=w165) -> ()  [unwired: 1 out]
    n60 = Unbundle By Name(w207) -> ("status"=w212:bool)
    n61 = Add(x=w122, y=w126) -> (x+y=w162:i32)
    n62 = Divide(x=w162, y=2) -> (x/y=w164:dbl)
    n63 = To Long Integer(number=w164) -> (32bit integer=w153:i32)
    n64 = Subtract(x=w153, y=w152) -> (x-y=w161:i32)
    n65 = In Range and Coerce(upper limit="Row max", x=w161, lower limit="Row min") -> (coerced(x)=w160:i32)  [unwired: 1 out]
    n66 = Add(x=w153, y=w152) -> (x+y=w154:i32)
    n67 = Add(x=w160, y=w149) -> (x+y=w159:i32)
    n68 = In Range and Coerce(upper limit="Row max", x=w154, lower limit="Row min") -> (coerced(x)=w150:i32)  [unwired: 1 out]
    n69 = Subtract(x=w150, y=w149) -> (x-y=w151:i32)
    n70 = In Range and Coerce(upper limit="Row max", x=w159, lower limit="Row min") -> (coerced(x)=w158:i32)  [unwired: 1 out]
    n71 = In Range and Coerce(upper limit="Row max", x=w151, lower limit="Row min") -> (coerced(x)=w148:i32)  [unwired: 1 out]
    n72 = while {
      tunnel: w127 -> [w240]
      tunnel: [w231] -> w123
      tunnel: [w241] -> w125
      tunnel: w146 -> [w243]
      tunnel: w144 -> [w245]
      tunnel: w158 -> [w232]
      tunnel: w160 -> [w233]
      tunnel: [w237] -> w117
      tunnel: "Pixel intensity\nthreshold" -> [w235]
      i -> [w234]
      stop <- w238 stop-if-true
      # "if true\nno TE found"
      # "camera 1"
      # "if there is a pixel\ndarker than the\ndark threshhold\nthen stop looking"
      # "row"
      # "image row"
      n73 = Add(x=w233, y=w234) -> (x+y=w231:i32)
      n74 = Index Array(array=w245, index (row)=w231) -> (element=w244:u8[])  [unwired: 1 in]
      n75 = Array Subset(array=w244, index=w240, length=w243) -> (w242:u8[])
      n76 = Array Max & Min(array=w242) -> (min value=w230:u8, min index (indices)=w236:i32)  [unwired: 2 out]
      n77 = Less Or Equal?(x=w230, y=w235) -> (x <= y?=w239:bool)
      n78 = Greater Or Equal?(x=w231, y=w232) -> (x >= y?=w237:bool)
      n79 = Or(x=w239, y=w237) -> (x .or. y?=w238:bool)
      n80 = Add(x=w236, y=w240) -> (x+y=w241:i32)
    }
    n81 = while {
      tunnel: w127 -> [w223]
      tunnel: [w214] -> w120
      tunnel: [w224] -> w121
      tunnel: w146 -> [w226]
      tunnel: w144 -> [w228]
      tunnel: w148 -> [w215]
      tunnel: w150 -> [w216]
      tunnel: [w220] -> w115
      tunnel: "Pixel intensity\nthreshold" -> [w218]
      i -> [w217]
      stop <- w221 stop-if-true
      # "if true\nno TE found"
      # "camera 1"
      # "if there is a pixel\ndarker than the\ndark threshhold\nthen stop looking"
      # "column subset"
      # "image row"
      n82 = Subtract(x=w216, y=w217) -> (x-y=w214:i32)
      n83 = Index Array(array=w228, index (row)=w214) -> (element=w227:u8[])  [unwired: 1 in]
      n84 = Array Subset(array=w227, index=w223, length=w226) -> (w225:u8[])
      n85 = Array Max & Min(array=w225) -> (min value=w229:u8, min index (indices)=w219:i32)  [unwired: 2 out]
      n86 = Less Or Equal?(x=w229, y=w218) -> (x <= y?=w222:bool)
      n87 = Less Or Equal?(x=w214, y=w215) -> (x <= y?=w220:bool)
      n88 = Or(x=w222, y=w220) -> (x .or. y?=w221:bool)
      n89 = Add(x=w219, y=w223) -> (x+y=w224:i32)
    }
    n90 = Bundle By Name(cluster="Rectangle", "Left"=w127, "Top"=w123, "Right"=w124, "Bottom"=w120) -> (w140:T1)
    n91 = Build Array(w127, w123, w124, w120) -> ()  [unwired: 1 out]
    n92 = Bundle By Name(cluster="Origin", "X"=w125, "Y"=w123) -> (w157:cluster{"X":i32, "Y":i32})
    n93 = call "IMAQ Overlay Text"("Text Color (black)"="Marker\nText color", "String"="T", "Origin"=w157, "Image"=w155) -> ("Image Out"=w141:T4)  [unwired: 4 in, 3 out]
    n94 = Bundle By Name(cluster="Origin", "X"=w121, "Y"=w120) -> (w142:cluster{"X":i32, "Y":i32})
    n95 = Add(x=w127, y=w124) -> (x+y=w139:i32)
    n96 = Add(x=w123, y=w120) -> (x+y=w134:i32)
    n97 = call "IMAQ Overlay Text"("Text Color (black)"="Marker\nText color", "String"="B", "Origin"=w142, "Image"=w141) -> ("Image Out"=w133:T4)  [unwired: 4 in, 3 out]
    n98 = call "IMAQ Overlay Rectangle"("Rectangle"=w140, "Image"=w133) -> ("Image Out"=w111:T4)  [unwired: 8 in, 1 out]
    n99 = Divide(x=w139, y=2) -> (x/y=w137:dbl)
    n100 = Divide(x=w134, y=2) -> (x/y=w136:dbl)
    n101 = To Long Integer(number=w137) -> (32bit integer=w129:i32)
    n102 = To Long Integer(number=w136) -> (32bit integer=w128:i32)
    n103 = case shown="True" "Acquire\ndata" {
      tunnel: w179 -> [_ w275]
      tunnel: w129 -> [_ w299]
      tunnel: [w268 w311] -> w194
      tunnel: w193 -> [_ w310]
      tunnel: w128 -> [_ w298]
      tunnel: [w268 w309] -> w192
      tunnel: w191 -> [_ w308]
      tunnel: w178 -> [_ w304]
      tunnel: [w268 w307] -> w190
      tunnel: w189 -> [_ w306]
      tunnel: [w269 w305] -> w187
      tunnel: w188 -> [_ w305]
      tunnel: w186 -> [_ w286]
      tunnel: w177 -> [_ w303]
      tunnel: [w267 w303] -> w184
      tunnel: w183 -> [_ w302]
      tunnel: [FALSE w301] -> w182
      tunnel: w127 -> [_ w297]
      tunnel: w126 -> [_ w296]
      tunnel: w125 -> [_ w295]
      tunnel: w123 -> [_ w294]
      tunnel: w124 -> [_ w293]
      tunnel: w122 -> [_ w292]
      tunnel: w121 -> [_ w291]
      tunnel: w120 -> [_ w290]
      tunnel: w119 -> [_ w289]
      tunnel: [w265 w287] -> w118
      tunnel: w117 -> [_ w285]
      tunnel: w116 -> [_ w284]
      tunnel: w115 -> [_ w283]
      frame False {
        w266 = 0
        n104 = call <userlib>:"Get date and time stub for end of file.vi"() -> ("date and time stub"=w269:string)
        n105 = Tick Count (ms)() -> (millisecond timer value=w267:u32)
        n106 = Initialize Array(w266, w266, w266) -> (w265:i32[][])
        n107 = Initialize Array(w266, w266) -> (w268:i32[])
      }
      frame True {
        # "y center"
        # "x center"
        n108 = Not(x=w286) -> (.not. x?=w274:bool)
        n109 = Not(x=w284) -> (.not. x?=w272:bool)
        n110 = Subtract(x=w304, y=w303) -> (x-y=w300:u32)
        n111 = Not(x=w285) -> (.not. x?=w273:bool)
        n112 = Not(x=w283) -> (.not. x?=w271:bool)
        n113 = Build Array (concatenate)(w308, w298) -> (w309:i32[])
        n114 = Build Array (concatenate)(w310, w299) -> (w311:i32[])
        n115 = Build Array(w274, w273, w272, w271) -> (w281:bool[])
        n116 = Build Array (concatenate)(w306, w304) -> (w307:u32[])
        n117 = Boolean To (0,1)(Boolean=w281) -> (0, 1=w280:i16[])
        n118 = Index Array(array=w280) -> (element #1=w279:i16, element #2=w278:i16, element #3=w277:i16, element #4=w276:i16)  [unwired: 4 in]
        n119 = And Array Elements(Boolean array=w281) -> (logical AND=w270:bool)
        n120 = Greater Or Equal?(x=w300, y=w302) -> (x >= y?=w301:bool)
        n121 = Boolean To (0,1)(Boolean=w270) -> (0, 1=w282:i16)
        n122 = Build Array(w275, w300, w299, w298, w282, w297, w296, w279, w295, w294, w278, w293, w292, w277, w291, w290, w276) -> (w288:u32[])
        n123 = Build Array (concatenate)(w289, w288) -> (w287:u32[][])
      }
    }
    n124 = And(x="save for a \ndesignated \nperiod", y=w182) -> (x .and. y?=w181:bool)
    n125 = Compound Arithmetic op=OR(w212, "stop", w181) -> (w213:bool)
    n126 = Bundle By Name(cluster="Origin", "X"=w129, "Y"=w128) -> (w132:cluster{"X":i32, "Y":i32})
    n127 = call "IMAQ Overlay Points"("Color"="Marker\nText color", "Point"=w132, "Image"=w111) -> ("Image Out"=w110:T4)  [unwired: 7 in, 1 out]
    n128 = call "IMAQ Overlay Rectangle"("Rectangle"=w108, "Image"=w110) -> ("Image Out"=w109:T4)  [unwired: 8 in, 1 out]
    "Image" <- w109
    "LIVE" <- TRUE
  }
  "X positions\ncamera 1\n(image \ncoordinates)" <- w53
  "Y positions camera 1 \n(image \ncoordinates)" <- w49
  "date stub assigned" <- w68
  n129 = call <vilib>:"IMAQdx Close Camera.vi"("error in"=w91, "Session In"=w92) -> ("error out"=w81:errorcluster)  [unwired: 9 out]
  n130 = Index Array(array=w39, index (col)=1) -> (element=w42:u32[])  [unwired: 1 in]
  n131 = call <vilib>:"General Error Handler.vi"("error in (no error)"=w81) -> ()  [unwired: 1 in, 14 out]
  n132 = Divide(x=w42, y=1000) -> (x/y=w59:dbl[])
  "time (s)" <- w59
  n133 = Build Cluster Array(w59, w49) -> (w72:cluster{dbl, i32}[])
  n134 = Bundle(w59, w49) -> (→"Y position vs time":cluster{dbl[], i32[]})  [unwired: 1 out]
  n135 = flat-sequence {
    tunnel: w81 -> [_]
    frame #0 {
      w328 = FALSE
      n136 = local write "Acquire\ndata"(w328) -> ()
      n137 = local write "LIVE"(w328) -> ()
    }
  }
  n138 = Array Max & Min(array=w59) -> (max value=w78:dbl)  [unwired: 3 out]
  n139 = Bundle(w59, w53) -> (→"X position vs time":cluster{dbl[], i32[]})  [unwired: 1 out]
  n140 = Array Size(array=w49) -> (size(s)=w77:i32)
  n141 = Build Cluster Array(w59, w53) -> (w73:cluster{dbl, i32}[])
  n142 = Build Cluster Array(w73, w72) -> (→"Multiplot":cluster{cluster{dbl, i32}[]}[])
  n143 = Divide(x=w77, y=w78) -> (x/y=→"FPS":dbl)
  n144 = Bundle(w53, w49) -> (→"trajectory":cluster{i32[], i32[]})  [unwired: 1 out]
  n145 = Index Array(array=w39, index (col)=w37) -> (element=w41:u32[])  [unwired: 1 in]
  n146 = while {
    tunnel: w59 -> [_]
    tunnel: w53 -> [_]
    tunnel: w49 -> [_]
    tunnel: [w329] -> w63
    tunnel: ["Experimental stub"] -> w71
    tunnel: [w332] -> w66
    tunnel: ["Experimental stub"] -> w64
    tunnel: ["save\nlast\nimage"] -> w62
    stop <- w334 stop-if-true
    n147 = call <userlib>:"make directory if it doesnt already exist.vi"("Path"="save path") -> ("created path"=w329:path)
    n148 = case shown="True" "always save\non stop\nimaging" {
      tunnel: [w338 w339] -> w332
      tunnel: "always save\non stop\nimaging" -> [_ w339]
      tunnel: "save data" -> [w338 _]
      frame False {
      }
      frame True {
      }
    }
    n149 = Compound Arithmetic op=OR("always save\non stop\nimaging", "stop no save", "save data") -> (w334:bool)
  }
  n150 = case shown="True" w62 {
    tunnel: w65 -> [_ w347]
    tunnel: w64 -> [_ w345]
    tunnel: w63 -> [_ w340]
    frame False {
    }
    frame True {
      n151 = call <userlib>:"Get date and time stub for end of file.vi"() -> ("date and time stub"=w343:string)
      n152 = Concatenate Strings(w345, "_last_image", w343, ".bmp") -> (w346:string)
      n153 = Build Path(base path=w340, name or relative path=w346) -> (appended path=w341:path)
      n154 = call-poly "IMAQ Write File 2"("File Path"=w341, "Image"=w347) -> ()  [unwired: 8 in, 2 out]
    }
  }
  n155 = Index Array(array=w41) -> (element=w40:u32)  [unwired: 1 in]
  n156 = Subtract(x=w41, y=w40) -> (x-y=w38:u32[])
  n157 = Increment(x=w38) -> (x+1=w36:u32[])
  n158 = Replace Array Subset(array=w39, new element=w36, index (col)=w37) -> (w2:u32[][])  [unwired: 1 in]
  n159 = Index Array(array=w2, index (col)=9) -> (element=w15:u32[])  [unwired: 1 in]
  n160 = Index Array(array=w2, index (col)=14) -> (element=w9:u32[])  [unwired: 1 in]
  n161 = Index Array(array=w2, index (col)=8) -> (element=w17:u32[])  [unwired: 1 in]
  n162 = Index Array(array=w2, index (col)=15) -> (element=w7:u32[])  [unwired: 1 in]
  n163 = Index Array(array=w2, index (col)=3) -> (element=w23:u32[])  [unwired: 1 in]
  n164 = Index Array(array=w2, index (col)=6) -> (element=w19:u32[])  [unwired: 1 in]
  n165 = Index Array(array=w2, index (col)=11) -> (element=w13:u32[])  [unwired: 1 in]
  n166 = Index Array(array=w2, index (col)=5) -> (element=w21:u32[])  [unwired: 1 in]
  n167 = Index Array(array=w2, index (col)=12) -> (element=w11:u32[])  [unwired: 1 in]
  n168 = Index Array(array=w2, index (col)=2) -> (element=w25:u32[])  [unwired: 1 in]
  n169 = Subtract(x=w25, y=w4) -> (x-y=w24:u32[])
  n170 = Subtract(x=w23, y=w5) -> (x-y=w22:u32[])
  n171 = Transpose 2D Array(2D array=w2) -> (transposed array=w1:u32[][])
  n172 = Subtract(x=w17, y=w4) -> (x-y=w16:u32[])
  n173 = Subtract(x=w15, y=w5) -> (x-y=w14:u32[])
  n174 = Subtract(x=w21, y=w4) -> (x-y=w20:u32[])
  n175 = Subtract(x=w19, y=w5) -> (x-y=w18:u32[])
  n176 = call <vilib>:"Histogram.vi"("intervals"="histogram \nbins", "X"=w53) -> ("Histogram Graph"=→"x position histogram":T2)  [unwired: 6 in, 3 out]
  n177 = call <vilib>:"Histogram.vi"("intervals"="histogram \nbins", "X"=w49) -> ("Histogram Graph"=→"y position histogram":T2)  [unwired: 6 in, 3 out]
  n178 = Subtract(x=w7, y=w5) -> (x-y=w6:u32[])
  n179 = Subtract(x=w11, y=w5) -> (x-y=w10:u32[])
  n180 = Subtract(x=w9, y=w4) -> (x-y=w8:u32[])
  n181 = Subtract(x=w13, y=w4) -> (x-y=w12:u32[])
  n182 = Build Array (concatenate)(w1, w24, w22, w20, w18, w16, w14, w12, w10, w8, w6) -> (w3:u32[][])
  n183 = case shown="True" w66 {
    tunnel: w71 -> [_ w354]
    tunnel: w63 -> [_ w353]
    tunnel: w68 -> [_ w350]
    tunnel: w3 -> [_ w349]
    frame False {
    }
    frame True {
      n184 = Transpose 2D Array(2D array=w349) -> (transposed array=w348:u32[][])
      n185 = Concatenate Strings(w354, w350, ".xls") -> (w352:string)
      n186 = Build Path(base path=w353, name or relative path=w352) -> (appended path=w351:path)
      n187 = stacked-sequence {
        tunnel: w351 -> [_ w358 _]
        tunnel: w348 -> [_ w357 _]
        frame #0 {
          "Saving" <- TRUE
        }
        frame #1 {
          n188 = call-poly <vilib>:"Write To Spreadsheet File.vi"("transpose? (no:F)"=FALSE, "format (%d)"="number\nformat (%.6f)", "2D data"=w357, "file path (dialog if empty)"=w358) -> ()  [unwired: 4 in, 1 out]
        }
        frame #2 {
          n189 = local write "Saving"(FALSE) -> ()
        }
      }
    }
  }
